vi "Different Types.vi"() -> ()   [LabVIEW 2017, in "Assertions.Tests.lvlib" / "Assert Greater Than.lvlib"]
uses:
  Assert Greater Than.lvlib
  src/Transparent Assertions/Constraints/Is Greater Than/Create.vi
  src/Transparent Assertions/Constraints/Is Greater Than/Is Greater Than.lvclass
  src/Transparent Assertions/Assertions/Assertions.lvlib
panel:
  out "error out":errorcluster
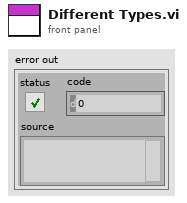
[diagram p1: front panel]
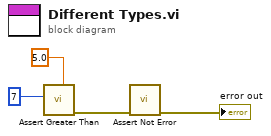
[diagram p0: block diagram]
diagram:
  n1 = call "Assert Greater Than.vi"("Expected"=5.0, "Actual"=7) -> ("error out"=w4:errorcluster)  [unwired: 9 in]
  n2 = call "Assert Not Error.vi"("error in (no error)"=w4) -> ("error out"=→"error out":errorcluster)  [unwired: 10 in]
